vi "PC Streaming Host with slow.vi"() -> ()   [LabVIEW 2012]
uses:
  <vilib>/userdefined/High Color/nirio_resource_hc.ctl
  hv cluster control.ctl
  <vilib>/FPGAPlugInAG/PXI-7951R/niLvFpga_Open_PXI-7951R.vi
  <vilib>/rvi/interface/common/dynamic/niFpgaDynamicAddResources.vi
  <vilib>/Utility/error.llb/Error Cluster From Error Code.vi
  <vilib>/rvi/errors/niLvFpgaAdjustHostInterfaceError.vi
  <vilib>/FPGAPlugInAG/Dynamic/niLvFpga_Close_Dynamic.vi
  <vilib>/rvi/interface/nirviOpenFPGA/nirviOpenFPGA.xnode
  FPGA Bitfiles/ModuDAQ_FPGATarget_TopLevelFPGAw8LE_8T5P+CgHwo4.lvbitx
  <vilib>/rvi/interface/nirviReadWriteControl/nirviReadWriteControl.xnode
  <vilib>/rvi/interface/nirviMethod/nirviMethod.xnode
  <vilib>/rvi/interface/nirviCloseFPGA/nirviCloseFPGA.xnode
  <vilib>/ptbypt/NI_PtbyPt.lvlib
  <vilib>/rvi/interface/Simulation/niFpgaSimulationCallBeginRW.vi
  Program Files/CAEN/HV/CAENHVWrapper/labview/CAENHVWrapper/CAENHVWrapper.lvlib
  NiFpgaLv.dll
  <vilib>/FPGAPlugInAG/Dynamic/niLvFpga_ReadFifo_Dynamic.vi
  <vilib>/rvi/errors/niLvFpgaMergeErrorWithErrorCode.vi
panel:
  in  "pressed stop by user after \nfile is fully written":bool
  out "Stop after file is fully written":bool
  out "fast loop stop":bool
  in  "Channel Cluster":T1={"det_type"=["", "", "", "", "", "", "", ""], "Serial numbers"=["", "", "", "", "", "", "", ""], "Sources"=["", "", "", "", "", "", "", ""], "Trigger level"=[4000, 4000, 4000, 4000, 4000, 4000, 4000, 4000], "Data Record On/Off"=[FALSE, FALSE, FALSE, FALSE, FALSE, FALSE, FALSE, FALSE, TRUE, FALSE, FALSE, FALSE, FALSE, FALSE, FALSE, TRUE], "Number of Channels"=8}
  in  "HV Cluster":T2={"HV Power On/Off"=[TRUE, TRUE], "Set Voltage"=["0", "0", "0", "0", "0", "0", "0", "0"], "HV Tolerance (%)"=1.0}
  out "created path":path
  out "File name":string
  out "Total Data Chunks to Write":dbl
  in  "Tab Control":T3(tab)
  in  "Write mode":bool
  out "directory exists - please wait":u8(slide)
  out "directory ok":bool
  in  "Write Enable":bool
  in  "File Path":path=path "Z:/Modulation/Raw_Data/combined"
  out "File Writing Progress (%)":dbl(slide) scale=0.0..100.0
  in  "Slow Control On":bool
  in  "Fast Data On":bool
  in  "Number of Files to Write":u32=1
  in  "IP Address of NIST Time Server":string(combo)="ntp1.nikhef.nl"
  in  "VISA resource name":refnum<visa-resource-name>="COM7"
  out "HV Power On/Off":bool[](array[boolean])
  in  "HV Tolerance (%)":dbl=1.0
  out "HV(V)":sgl[](array[numeric])
  in  "IP adress HV2":string="1_0_0"
  in  "IP adress HV1":string="0_0_0"
  out "error HV":errorcluster
  out "Set Voltage":string[](array[string])=["0", "0", "0", "0", "0", "0", "0", "0"]
  out "Current(uA)":sgl[](array[numeric])
  in  "General Cluster":cluster{"Location":i16}={"Location"=1} {"Location" items=["Purdue", "NIKHEF", "Zurich", "???"]}
  in  "PXI address":T4="RIO0" caption="RIO Device"
  in  "det_type":string[](array[combo])=["NaI(Tl)", "NaI(Tl)", "NaI(Tl)", "NaI(Tl)", "NaI(Tl)", "NaI(Tl)", "NaI(Tl)", "NaI(Tl)"]
  in  "Serial numbers":string[](array[combo])=["SBJ593", "SBJ592", "SBJ590", "SBJ591", "SBJ588", "SBJ589", "SBJ586", "Other"]
  in  "Sources":string[](array[combo])=["Background", "Background", "Ti-44", "Ti-44", "Co-60", "Co-60", "Cs-137", "Cs-137"]
  in  "Trigger level":i16[](array[numeric])=[2000, 2000, 1000, 1000, 2000, 2000, 2000, 2000] caption="Trigger"
  in  "Data Record \nOn/Off":bool[](array[boolean])=[TRUE, TRUE, TRUE, TRUE, TRUE, TRUE, TRUE, TRUE]
  in  "Testpulse Cluster":T5={"Master Pulser On/Off"=FALSE, "Testpulse Turnaround Time (samples)"=14, "Pulse Separation (samples)"=0, "Pulse duration (samples)"=0}
  out "Samples per Data Chunk":u32
  in  "DAQ Info Cluster":T6={"Data Chunks per File"=1000, "Samples per Waveform"=95, "Pretrigger Samples"=15, "circular buffer length (samples)"=1000, "Waveforms per Data Chunk"=5000} {"Waveforms per Data Chunk" format="%.2p"}
  out "Average Throughput":dbl(graph)
  out "Loop Time":u32
  out "Inst. Throughput":dbl format="%#_6p"
  out "Elements in FIFO":u32(graph)
  out "FIFO Overflow":bool
  out "Current Chunk":u32
  out "Current File":i32
  out "Waveform Graph":dynamicdata(graph)
  out "Channel number displayed":i16=-1
  in  "Arduino read \nrate (Hz)":dbl=1.0
  out "Slow time":u64
  out "data":dbl[](array[numeric])
  in  "XON Character":u8=17 format="%.0x"
  in  "XOFF Character":u8=19 format="%.0x"
  out "Slow Cluster":T7
  out "read buffer":string
  out "Bad sensor?":string
  in  "Max Slow Entries per File":i32=86400
  out "Current Slow File":i32
  out "Current Slow Entry":i32
  out "Sensor out of bounds":bool
  out "Temperature":dbl(graph)
  out "Pressure":dbl(graph)
  out "magnetic field y coordinate":dbl(graph)
  out "total magnetic field":dbl(graph)
  out "magnetic field z coordinate":dbl(graph)
  out "magnetic field x coordinate":dbl(graph)
  out "humidity":dbl(graph)
  out "XML String":string
  out "Slow XML":string
  out "error out":errorcluster
  out "NIST Time":u64
  out "NIST Time Failed to Read":bool
  in  "Minutes to wait":u32=5 min=3
  out "UTC format":bool=TRUE
  out "FPGA Timestamp":u64
  out "Stopped":bool
  in  "stop":bool
  # "Channel 0"
  # "Channel 1"
  # "Channel 2"
  # "Channel 3"
  # "Channel 4"
  # "Channel 5"
  # "Channel 6"
  # "Channel 7"
  # "Write continuously"
  # "Write finite number of files"
  # "Program will stop when number of Files to Write is Complete OR if stop is pressed."
  # "These parameters are set by the set_shutdown_HV vi!"
  # "Channel 0"
  # "Channel 1"
  # "Channel 2"
  # "Channel 3"
  # "Channel 4"
  # "Channel 5"
  # "Channel 6"
  # "Channel 7"
  # "Channel 0"
  # "Channel 1"
  # "Channel 2"
  # "Channel 3"
  # "Channel 4"
  # "Channel 5"
  # "Channel 6"
  # "Channel 7"
  # "TODO: Make this look like the \"detectors\" tab"
  # "Waveform/Data Chunk information"
  # "To compare directly on a scope: Horizontal scale: 200 ns/div Vertical scale: ~100 mV/div If 15 pretriggers, delay = 700 ns"
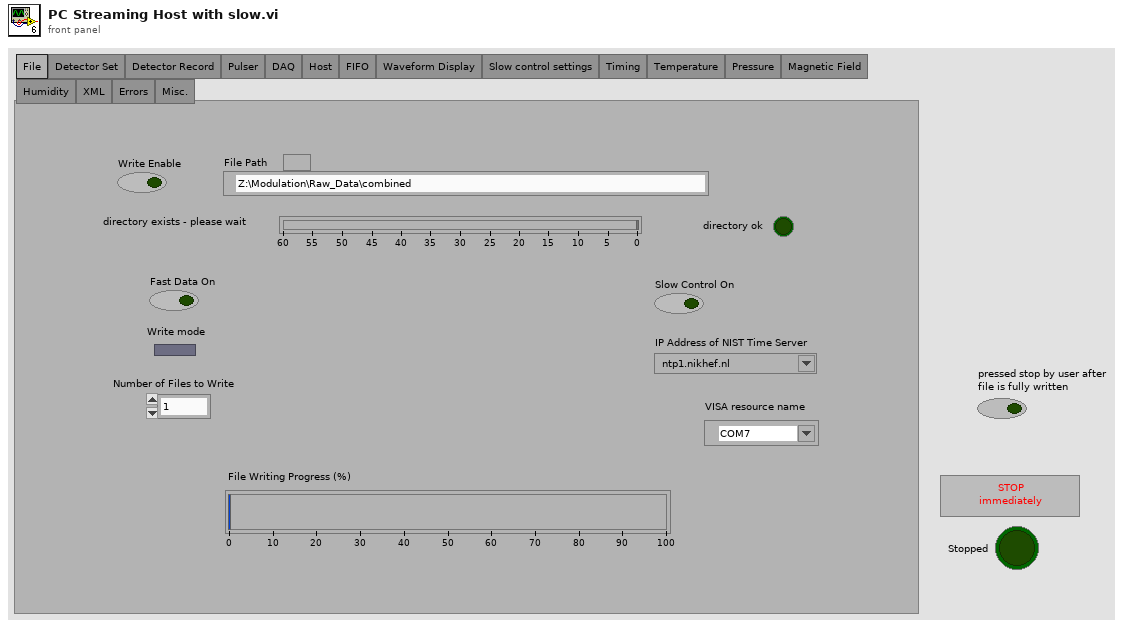
[diagram p1: front panel]
types:
  T1 = cluster{"det_type":string[], "Serial numbers":string[], "Sources":string[], "Trigger level":i16[], "Data Record On/Off":bool[], "Number of Channels":u8}
  T2 = typedef "hv cluster control.ctl" = cluster{"HV Power On/Off":bool[], "Set Voltage":string[], "HV Tolerance (%)":dbl}
  T3 = enum32{"File", "Detector Set", "Detector Record", "Pulser", "DAQ", "Host", "FIFO", "Waveform Display", "Slow control settings", "Timing", "Temperature", "Pressure", "Magnetic Field", "Humidity", "XML", "Errors", "Misc."}
  T4 = typedef "nirio_resource_hc.ctl" = tag
  T5 = cluster{"Master Pulser On/Off":bool, "Testpulse Turnaround Time (samples)":u32, "Pulse Separation (samples)":u32, "Pulse duration (samples)":u32}
  T6 = cluster{"Data Chunks per File":u32, "Samples per Waveform":u32, "Pretrigger Samples":u32, "circular buffer length (samples)":u32, "Waveforms per Data Chunk":u32}
  T7 = cluster{"Arduino \nParameters":dbl, "Total Number of \nSlow Parameters":i32, "UTC format?":bool, "Sensor Upper \nbounds":i32[], "Sensor Lower \nbounds":i32[], "Descriptions":string[], "datanames":string[]}
  T8 = cluster{"Arduino Parameters":dbl, "Total Number of Slow Parameters":i32, "UTC format?":bool, "Sensor Upper bounds":i32[], "Sensor Lower bounds":i32[], "Descriptions":string[], "datanames":string[]}
  T9 = enum16{"open", "replace", "create", "open or create", "replace or create", "replace or create with confirmation"}
  T10 = enum16{"big-endian, network order", "native, host order", "little-endian"}
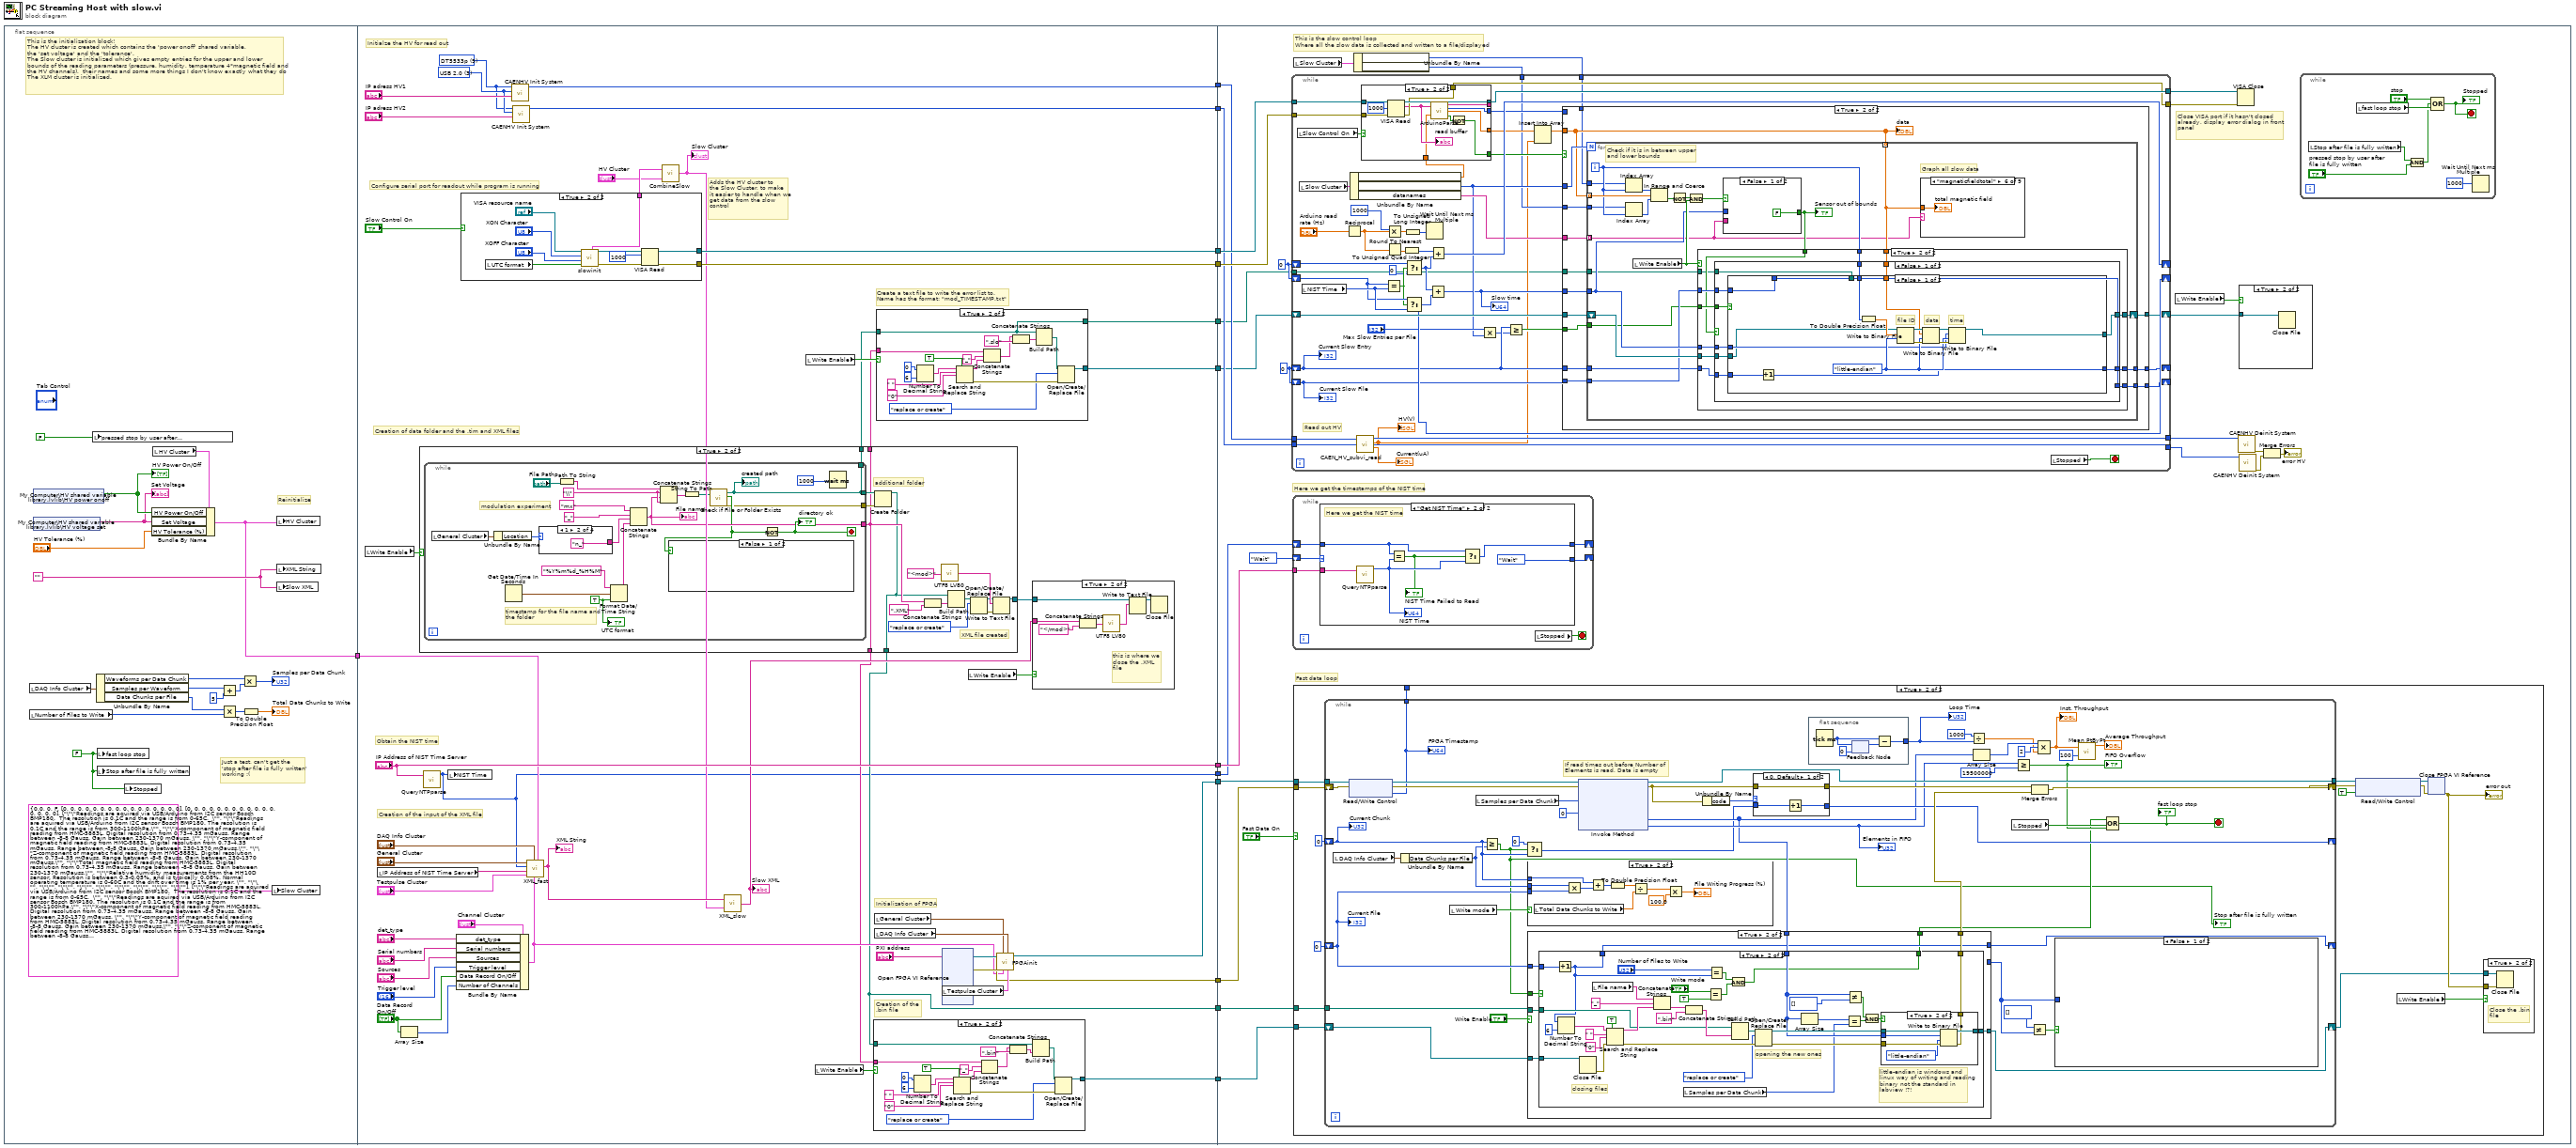
[diagram p0: block diagram]
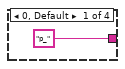
[diagram p7: hidden frame]
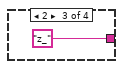
[diagram p8: hidden frame]
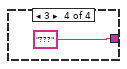
[diagram p9: hidden frame]
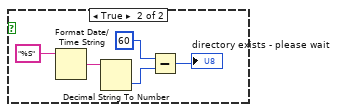
[diagram p10: hidden frame]
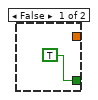
[diagram p11: hidden frame]
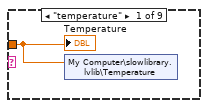
[diagram p13: hidden frame]
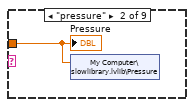
[diagram p14: hidden frame]
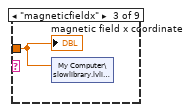
[diagram p15: hidden frame]
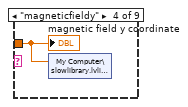
[diagram p16: hidden frame]
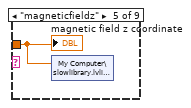
[diagram p17: hidden frame]
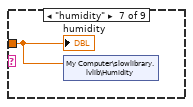
[diagram p18: hidden frame]
diagram:
  n1 = flat-sequence {
    tunnel: [w15] -> w2
    tunnel: ["IP Address of NIST Time Server"] -> w13
    tunnel: [w58] -> w12
    tunnel: [w57] -> w11
    tunnel: [w53] -> w10
    tunnel: [w52] -> w9
    tunnel: [w51] -> w8
    tunnel: [w42] -> w7
    tunnel: [w41] -> w6
    tunnel: [w40] -> w5
    tunnel: [w36] -> w4
    tunnel: [w35] -> w3
    tunnel: w2 -> [w34]
    tunnel: [w33] -> w1
    tunnel: w13 -> [w195]
    tunnel: w12 -> [w186]
    tunnel: w11 -> [w185]
    tunnel: w10 -> [w182]
    tunnel: w9 -> [w184]
    tunnel: w8 -> [w183]
    tunnel: w7 -> [w181]
    tunnel: w6 -> [w180]
    tunnel: w5 -> [w179]
    tunnel: w4 -> [w177]
    tunnel: w3 -> [w176]
    tunnel: w1 -> [w175]
    frame #0 {
      w14 = FALSE ("fast loop stop")
      w31 = ""
      # "Just a test, can't get the \n'stop after file is fully written'\nworking :("
      # "This is the initialization block!\nThe HV cluster is created which contains the 'power onoff' shared variable, \nthe 'set voltage' and the 'tolerance'.\nThe Slow cluster is initialized which gives empty entries for the upper and lower\nbounds of the reading parameters (pressure, humidity, temperature 4*magnetic field and\nthe HV channels),  their names and some more things I don't know exactly what they do\nThe XLM cluster is initialized."
      # "Reinitialize"
      n2 = local read "DAQ Info Cluster"() -> (w27:T6)
      n3 = local read "Number of Files to Write"() -> (w22:u32)
      n4 = shared-variable "My Computer\\HV shared variable library.lvlib\\HV power onoff"() -> (w17:bool[])  [unwired: 1 in, 1 out]
      "HV Power On/Off" <- w17
      n5 = shared-variable "My Computer\\HV shared variable library.lvlib\\HV voltage set"() -> (w16:string[])  [unwired: 1 in, 1 out]
      "Set Voltage" <- w16
      n6 = local write "pressed stop by user after \nfile is fully written"(FALSE ("stop 2")) -> ()
      n7 = Unbundle By Name(w27) -> ("Waveforms per Data Chunk"=w19:u32, "Samples per Waveform"=w20:u32, "Data Chunks per File"=w21:u32)
      n8 = local write "fast loop stop"(w14) -> ()
      n9 = local write "Stop after file is fully written"(w14) -> ()
      n10 = local write "Stopped"(w14) -> ()
      n11 = local read "HV Cluster"() -> (w30:T2)
      n12 = Bundle By Name(cluster=w30, "HV Power On/Off"=w17, "Set Voltage"=w16, "HV Tolerance (%)"="HV Tolerance (%)") -> (w15:T2)
      n13 = Add(x=w20, y=u32 5) -> (x+y=w24:u32)
      n14 = Multiply(x=w21, y=w22) -> (x*y=w26:u32)
      n15 = Multiply(x=w19, y=w24) -> (x*y=→"Samples per Data Chunk":u32)
      n16 = To Double Precision Float(number=w26) -> (double precision float=→"Total Data Chunks to Write":dbl)
      n17 = local write "Slow Cluster"(T8 {"Arduino Parameters"=0.0, "Total Number of Slow Parameters"=0, "UTC format?"=FALSE, "Sensor Upper bounds"=[0, 0, 0, 0, 0, 0, 0, 0, 0, 0, 0, 0, 0, 0, 0, 0], "Sensor Lower bounds"=[0, 0, 0, 0, 0, 0, 0, 0, 0, 0, 0, 0, 0, 0, 0, 0], "Descriptions"=["\"\"Readings are aquired via USB/Arduino from I2C sensor Bosch BMP180.  The resolution is 0.1C and the range is from 0-65C.  \"", "\"\"Readings are aquired via USB/Arduino from I2C sensor Bosch BMP180. The resolution is 0.1C and the range is from 300-1100hPa.\"", "\"\"X-component of magnetic field reading from HMC-5883L. Digital resolution from 0.73-4.35 mGauss. Range between -8-8 Gauss. Gain between 230-1370 mGauss. \"", "\"\"Y-component of magnetic field reading from HMC-5883L. Digital resolution from 0.73-4.35 mGauss. Range between -8-8 Gauss. Gain between 230-1370 mGauss.\"", "\"\"Z-component of magnetic field reading from HMC-5883L. Digital resolution from 0.73-4.35 mGauss. Range between -8-8 Gauss. Gain between 230-1370 mGauss.\"", "\"\"Total magnetic field reading from HMC-5883L. Digital resolution from 0.73-4.35 mGauss. Range between -8-8 Gauss. Gain between 230-1370 mGauss.\"", "\"\"Relative humidity measurements from the HH10D sensor. Resolution is between 0.3-0.05%, and is typically 0.08%. Normal operating temperature is 0-60C and the drift over time is 1% per year. \"", "\"\"", "\"\"", "\"\"", "\"\"", "\"\"", "\"\"", "\"\"", "\"\"", "\"\""], "datanames"=["\"\"Readings are aquired via USB/Arduino from I2C sensor Bosch BMP180.  The resolution is 0.1C and the range is from 0-65C.  \"", "\"\"Readings are aquired via USB/Arduino from I2C sensor Bosch BMP180. The resolution is 0.1C and the range is from 300-1100hPa.\"", "\"\"X-component of magnetic field reading from HMC-5883L. Digital resolution from 0.73-4.35 mGauss. Range between -8-8 Gauss. Gain between 230-1370 mGauss. \"", "\"\"Y-component of magnetic field reading from HMC-5883L. Digital resolution from 0.73-4.35 mGauss. Range between -8-8 Gauss. Gain between 230-1370 mGauss.\"", "\"\"Z-component of magnetic field reading from HMC-5883L. Digital resolution from 0.73-4.35 mGauss. Range between -8-8 Gauss. Gain between 230-1370 mGauss.\"", "\"\"Total magnetic field reading from HMC-5883L. Digital resolution from 0.73-4.35 mGauss. Range between -8-8 Gauss. Gain between 230-1370 mGauss.\"", "\"\"Relative humidity measurements from the HH10D sensor. Resolution is between 0.3-0.05%, and is typically 0.08%. Normal operating temperature is 0-60C and the drift over time is 1% per year. \"", "\"\"", "\"\"", "\"\"", "\"\"", "\"\"", "\"\"", "\"\"", "\"\"", "\"\""]} ("Cluster")) -> ()
      n18 = local write "HV Cluster"(w15) -> ()
      n19 = local write "XML String"(w31) -> ()
      n20 = local write "Slow XML"(w31) -> ()
    }
    frame #1 {
      w60 = 3 items=["TCP/IP"=0, "HS CAENET"=2, "USB 2.0"=3, "CONET Optical Link"=4, "USB VCP"=5] ("LinkType")
      w59 = u32 9 items=["SY1527", "SY2527", "SY4527", "SY5527", "N568", "V65XX", "N1470", "V8100", "", "DT5533p"] ("system")
      # "Creation of the \n.bin file"
      # "Obtain the NIST time"
      # "Adds the HV cluster to\nthe Slow Cluster, to make\nit easier to handle when we\nget data from the slow\ncontrol"
      # "Initialization of FPGA"
      # "Initialze the HV for read out"
      # "Create a text file to write the error list to.  \nName has the format: \"mod_TIMESTAMP.txt\""
      # "Creation of the input of the XML file"
      # "Configure serial port for readout while program is running"
      # "Creation of data folder and the .tim and XML files"
      n21 = local read "Write Enable"() -> (w81:bool)
      n22 = local read "IP Address of NIST Time Server"() -> (w72:string)
      n23 = Array Size(array="Data Record \nOn/Off") -> (size(s)=w70:i32)
      n24 = case shown="True" w81 {
        tunnel: [_ w143] -> w54
        tunnel: [_ w135] -> w56
        tunnel: [_ w133] -> w43
        tunnel: [_ w133] -> w37
        tunnel: [_ w132] -> w36
        frame False {
        }
        frame True {
          # "XML file created"
          # "additional folder"
          n25 = while {
            tunnel: [w146] -> w144
            tunnel: [w148] -> w145
            tunnel: [w148] -> w143
            tunnel: [w153] -> w133
            stop <- w158 stop-if-true
            w154 = "\\" ("string")
            w161 = TRUE ("UTC format")
            # "modulation experiment"
            # "timestamp for the file name and the folder"
            n26 = local read "General Cluster"() -> (w151:cluster{"Location":i16})
            n27 = Unbundle By Name(w151) -> ("Location"=w150:i16)
            n28 = Get Date/Time In Seconds() -> (seconds since 1Jan1904=w162:timestamp)
            n29 = case shown="1" w150 {
              tunnel: ["p_" ("string") "n_" ("string") "z_" ("string") "???"] -> w152
              frame 0, Default {
              }
              frame 1 {
              }
              frame 2 {
              }
              frame 3 {
              }
            }
            n30 = Path To String(path="File Path") -> (string=w164:string)
            n31 = Format Date/Time String(time format string (%c)="%Y%m%d_%H%M", seconds (now)=w162, UTC format=w161) -> (date/time string=w155:string)
            n32 = Concatenate Strings("mx" ("string"), "_" ("string"), w152, w155) -> (w153:string)
            "File name" <- w153
            n33 = Concatenate Strings(w164, w154, w153, w154) -> (w165:string)
            n34 = String To Path(string=w165) -> (path=w149:path)
            n35 = call <vilib>:"Check if File or Folder Exists.vi"("path"=w149) -> ("error out"=w146:errorcluster, "file or folder exists?"=w147:bool, "dup path"=w148:path)  [unwired: 8 in]
            "created path" <- w148
            n36 = case shown="False" w147 {
              frame False {
              }
              frame True {
                n37 = Format Date/Time String(time format string (%c)="%S") -> (date/time string=w173:string)  [unwired: 2 in]
                n38 = Decimal String To Number(string=w173) -> (number=w171:i32)  [unwired: 2 in, 1 out]
                n39 = Subtract(x=60, y=w171) -> (x-y=→"directory exists - please wait":i32)
              }
            }
            n40 = Not(x=w147) -> (.not. x?=w158:bool)
            "directory ok" <- w158
            n41 = Wait (ms)(milliseconds to wait=1000) -> ()  [unwired: 1 out]
            "UTC format" <- w161
          }
          n42 = Create Folder(path (use dialog)=w145, error in=w144) -> (created path=w132:path)  [unwired: 1 in, 2 out]
          n43 = Concatenate Strings(w133, ".XML" ("substring (\"\")")) -> (w139:string)
          n44 = call "UTF8 LV80.vi"("text"="<mod>") -> ("utf-8 text out"=w142:string)
          n45 = Build Path(base path=w132, name or relative path=w139) -> (appended path=w138:path)
          n46 = Open/Create/Replace File(file path (use dialog)=w138, operation (0:open)=T9."replace or create") -> (refnum out=w141:refnum<file>, error out=w140:errorcluster)  [unwired: 4 in, 1 out]
          n47 = Write to Text File(file (use dialog)=w141, text=w142, error in=w140) -> (refnum out=w135:refnum<file>)  [unwired: 1 in, 2 out]
        }
      }
      n48 = call "QueryNTPparse.vi"("IP Address of NIST Server"="IP Address of NIST Time Server") -> ("NTP Time"=w33:u64)  [unwired: 1 in, 2 out]
      n49 = local write "NIST Time"(w33) -> ()
      n50 = Bundle By Name(cluster="Channel Cluster", "det_type"="det_type", "Serial numbers"="Serial numbers", "Sources"="Sources", "Trigger level"="Trigger level", "Data Record On/Off"="Data Record \nOn/Off", "Number of Channels"=w70) -> (w39:T1)
      n51 = case shown="True" "Slow Control On" {
        tunnel: [_ w131] -> w58
        tunnel: [_ w130] -> w57
        tunnel: [_ w122] -> w80
        frame False {
        }
        frame True {
          n52 = local read "UTC format"() -> (w125:bool)
          n53 = call "slowinit.vi"("UTC format"=w125, "XOFF Character"="XOFF Character", "XON Character"="XON Character", "VISA resource name"="VISA resource name") -> ("error IO"=w123:errorcluster, "VISA resource name out"=w124:refnum<visa-resource-name>, "Slow Cluster"=w122:T8)  [unwired: 5 in]
          n54 = VISA Read(VISA resource name=w124, byte count=u32 1000, error in (no error)=w123) -> (VISA resource name out=w131:refnum<visa-resource-name>, error out=w130:errorcluster)  [unwired: 2 out]
        }
      }
      n55 = call "CAENHV Init System.vi"("Arg"="IP adress HV1", "LinkType"=w60, "system"=w59) -> ("handle"=w52:i32)  [unwired: 7 in, 1 out]
      n56 = call "CAENHV Init System.vi"("Arg"="IP adress HV2", "LinkType"=w60, "system"=w59) -> ("handle"=w51:i32)  [unwired: 7 in, 1 out]
      n57 = call "XML_fast.vi"("HV Cluster"=w34, "Channel Cluster"=w39, "DAQ Info Cluster"="DAQ Info Cluster", "Testpulse Cluster"="Testpulse Cluster", "IP Address of NIST Time Server"=w72, "NIST Time"=w33, "General Cluster"="General Cluster") -> ("XML String"=w75:string)  [unwired: 4 in]
      "XML String" <- w75
      n58 = call "CombineSlow.vi"("HV Cluster"="HV Cluster", "Slow Cluster"=w80) -> ("Slow Cluster 2"=w38:T8)
      "Slow Cluster" <- w38
      n59 = call "XML_slow.vi"("Slow Cluster"=w38, "Input String"=w75) -> ("Output String"=w76:string)
      "Slow XML" <- w76
      n60 = local read "Write Enable"() -> (w55:bool)
      n61 = local read "Write Enable"() -> (w44:bool)
      n62 = case shown="True" w44 {
        tunnel: [_ w91] -> w42
        tunnel: w37 -> [_ w83]
        tunnel: w36 -> [_ w82]
        frame False {
        }
        frame True {
          n63 = Number To Decimal String(number=0, width (-)=i16 6) -> (decimal integer string=w98:string)
          n64 = Search and Replace String(replace all?=TRUE ("replace all? (F)"), input string=w98, search string=" ", replace string="0" ("replace string (\"\")")) -> (result string=w88:string, error out=w93:errorcluster)  [unwired: 4 in, 2 out]
          n65 = Concatenate Strings(w83, "_" ("string"), w88) -> (w86:string)
          n66 = Concatenate Strings(w86, ".bin" ("substring (\"\")")) -> (w90:string)
          n67 = Build Path(base path=w82, name or relative path=w90) -> (appended path=w94:path)
          n68 = Open/Create/Replace File(file path (use dialog)=w94, error in=w93, operation (0:open)=T9."replace or create") -> (refnum out=w91:refnum<file>)  [unwired: 3 in, 2 out]
        }
      }
      n69 = local read "General Cluster"() -> (w47:cluster{"Location":i16})
      n70 = local read "DAQ Info Cluster"() -> (w48:T6)
      n71 = case shown="True" w55 {
        tunnel: [_ w108] -> w53
        tunnel: w43 -> [_ w100]
        tunnel: w54 -> [_ w99]
        tunnel: [_ w99] -> w35
        frame False {
        }
        frame True {
          n72 = Number To Decimal String(number=0, width (-)=i16 6) -> (decimal integer string=w115:string)
          n73 = Search and Replace String(replace all?=TRUE ("replace all? (F)"), input string=w115, search string=" ", replace string="0" ("replace string (\"\")")) -> (result string=w105:string, error out=w110:errorcluster)  [unwired: 4 in, 2 out]
          n74 = Concatenate Strings(w100, "_" ("string"), w105) -> (w103:string)
          n75 = Concatenate Strings(w103, ".slo" ("substring (\"\")")) -> (w107:string)
          n76 = Build Path(base path=w99, name or relative path=w107) -> (appended path=w111:path)
          n77 = Open/Create/Replace File(file path (use dialog)=w111, error in=w110, operation (0:open)=T9."replace or create") -> (refnum out=w108:refnum<file>)  [unwired: 3 in, 2 out]
        }
      }
      n78 = local read "Testpulse Cluster"() -> (w46:T5)
      n79 = xnode "Open FPGA VI Reference"("resource name"="PXI address") -> ("FPGA VI Reference Out"=w50:refnum<k20>, "error out"=w49:errorcluster)  [unwired: 1 in]
      n80 = local read "Write Enable"() -> (w63:bool)
      n81 = call "FPGAinit.vi"("Testpulse Cluster"=w46, "DAQ Info Cluster"=w48, "Channel Cluster"=w39, "General Cluster"=w47, "error in"=w49, "FPGA VI Reference In"=w50) -> ("error out"=w40:errorcluster, "FPGA VI Reference Out"=w41:refnum<k20>)  [unwired: 4 in]
      n82 = case shown="True" w63 {
        tunnel: w56 -> [_ w121]
        tunnel: w76 -> [_ w116]
        frame False {
        }
        frame True {
          # "this is where we close the .XML file"
          n83 = Concatenate Strings(w116, "</mod>" ("string")) -> (w117:string)
          n84 = call "UTF8 LV80.vi"("text"=w117) -> ("utf-8 text out"=w120:string)
          n85 = Write to Text File(file (use dialog)=w121, text=w120) -> (refnum out=w119:refnum<file>)  [unwired: 2 in, 2 out]
          n86 = Close File(refnum=w119) -> ()  [unwired: 1 in, 2 out]
        }
      }
    }
    frame #2 {
      w187 = 0
      w178 = u64 0
      # "This is the slow control loop\nWhere all the slow data is collected and written to a file/displayed"
      # "Fast data loop"
      # "Close VISA port if it hasn't closed already, display error dialog in front panel"
      # "Here we get the timestamps of the NIST time"
      n87 = while {
        shift-right: [w560] -> _
        shift-left: enum16{"Wait", "Get NIST Time", "Write"}."Wait" -> [w561]
        shift-right: [w559] -> _
        shift-left: w175 -> [w558]
        tunnel: w195 -> [w557]
        stop <- w556 stop-if-true
        n88 = case shown="\"Get NIST Time\"" w561 {
          tunnel: [w564 enum16{"Wait", "Get NIST Time", "Write"}."Wait"] -> w560
          tunnel: [w563 w579] -> w559
          tunnel: w558 -> [w563 w576]
          tunnel: w557 -> [_ w575]
          frame "Wait", Default {
            # "First we wait 'minutes to wait' and proceed with Getting the NIST time\nthis is necessary to see a  drift, if it is there, between the PFGA and NIST time"
            n89 = while {
              tunnel: [enum16{"Wait", "Get NIST Time", "Write"}."Get NIST Time"] -> w564
              tunnel: "Minutes to wait" -> [w566]
              i -> [w569]
              stop <- w570 stop-if-true
              n90 = local read "Stopped"() -> (w568:bool)
              n91 = Multiply(x=60, y=w566) -> (x*y=w565:u32)
              n92 = Wait Until Next ms Multiple(millisecond multiple=u32 1000 ("y")) -> ()  [unwired: 1 out]
              n93 = Greater Or Equal?(x=w569, y=w565) -> (x >= y?=w571:bool)
              n94 = Or(x=w571, y=w568) -> (x .or. y?=w570:bool)
            }
          }
          frame "Get NIST Time" {
            # "Here we get the NIST time"
            n95 = call "QueryNTPparse.vi"("IP Address of NIST Server"=w575) -> ("NTP Time"=w578:u64)  [unwired: 1 in, 2 out]
            "NIST Time" <- w578
            n96 = Equal?(x=w576, y=w578) -> (x = y?=w577:bool)
            "NIST Time Failed to Read" <- w577
            n97 = Select(t=w576, s=w577, f=w578) -> (s? t:f=w579:u64)
          }
        }
        n98 = local read "Stopped"() -> (w556:bool)
      }
      n99 = local read "Slow Cluster"() -> (w199:T7)
      n100 = case shown="True" "Fast Data On" {
        tunnel: [_ w402] -> _
        tunnel: w181 -> [_ w398]
        tunnel: w180 -> [_ w397]
        tunnel: w179 -> [_ w396]
        tunnel: w177 -> [_ w395]
        frame False {
        }
        frame True {
          n101 = while {
            shift-right: [w442] -> w404
            shift-left: w396 -> [w431]
            shift-right: [w438] -> _
            shift-left: u32 0 -> [w435]
            shift-right: [w423] -> _
            shift-left: 0 ("number") -> [w424]
            shift-right: [w439] -> w406
            shift-left: w398 -> [w440]
            tunnel: [w456] -> w401
            tunnel: [w428] -> w402
            tunnel: w397 -> [w417]
            tunnel: w395 -> [w415]
            stop <- w425 stop-if-true
            # "If read times out before Number of Elements is read, Data is empty"
            n102 = local read "DAQ Info Cluster"() -> (w419:T6)
            n103 = xnode "Read/Write Control"("FPGA VI Reference In"=w417, "error in"=w431) -> ("FPGA VI Reference Out"=w430:refnum<k20>, "error out"=w429:errorcluster, "Timestamp"=w428:u64)
            "FPGA Timestamp" <- w428
            n104 = Unbundle By Name(w419) -> ("Data Chunks per File"=w418:u32)
            n105 = local read "Write mode"() -> (w432:bool)
            n106 = local read "Samples per Data Chunk"() -> (w416:u32)
            n107 = Greater Or Equal?(x=w435, y=w418) -> (x >= y?=w412:bool)
            "Stop after file is fully written" <- w412
            n108 = Select(t=u32 0, s=w412, f=w435) -> (s? t:f=w414:u32)
            n109 = case shown="True" w432 {
              tunnel: w424 -> [_ w475]
              tunnel: w435 -> [_ w473]
              tunnel: w418 -> [_ w466]
              frame False {
              }
              frame True {
                n110 = local read "Total Data Chunks to Write"() -> (w470:dbl)
                n111 = Multiply(x=w466, y=w475) -> (x*y=w474:u32)
                n112 = Add(x=w473, y=w474) -> (x+y=w472:u32)
                n113 = To Double Precision Float(number=w472) -> (double precision float=w471:dbl)
                n114 = Divide(x=w471, y=w470) -> (x/y=w468:dbl)
                n115 = Multiply(x=w468, y=100.0) -> (x*y=→"File Writing Progress (%)":dbl)
              }
            }
            n116 = xnode "Invoke Method"("FPGA VI Reference In"=w430, "error in"=w429, "Number of Elements"=w416, "Timeout (ms)"=0) -> ("FPGA VI Reference Out"=w456:refnum<k20>, "error out"=w453:errorcluster, "Data"=w433:i16[], "Elements Remaining"=w434:u32)
            "Elements in FIFO" <- w434
            n117 = case shown="True" "Write Enable" {
              tunnel: w433 -> [w482 w488]
              tunnel: [w482 _] -> w422
              tunnel: w412 -> [_ w492]
              tunnel: [_ w491] -> w441
              tunnel: [w483 w490] -> w439
              tunnel: w440 -> [w483 w489]
              tunnel: w424 -> [w481 w487]
              tunnel: [w481 w486] -> w423
              tunnel: [FALSE w485] -> w413
              tunnel: w415 -> [_ w484]
              frame False {
              }
              frame True {
                n118 = case shown="True" w492 {
                  tunnel: w488 -> [w496 w521]
                  tunnel: [w495 w523] -> w491
                  tunnel: w489 -> [w500 w536]
                  tunnel: [w499 w529] -> w490
                  tunnel: w487 -> [w494 w508]
                  tunnel: [w494 w507] -> w486
                  tunnel: [FALSE w510] -> w485
                  tunnel: w484 -> [_ w509]
                  frame False {
                    # "binary writing will write 0 if there is no data"
                    n119 = Not Equal?(x=w496, y=i16[] []) -> (x != y?=w497:bool)
                    n120 = case shown="True" w497 {
                      tunnel: w500 -> [w501 w506]
                      tunnel: [w501 w505] -> w499
                      tunnel: [_ w504] -> w495
                      tunnel: w496 -> [_ w502]
                      frame False {
                      }
                      frame True {
                        n121 = Write to Binary File(file (use dialog)=w506, data=w502, 9:T10."little-endian" ("byte order (0:big-endian, network order)")) -> (refnum out=w505:refnum<file>, error out=w504:errorcluster)  [unwired: 3 in, 1 out]
                      }
                    }
                  }
                  frame True {
                    # "little-endian is windows and linux way of writing and reading binary not the standard in labview !?!"
                    # "opening the new ones"
                    # "closing files"
                    n122 = Increment(x=w508) -> (x+1=w507:i32)
                    n123 = Number To Decimal String(number=w507, width (-)=i16 6) -> (decimal integer string=w538:string)
                    n124 = Close File(refnum=w536) -> (error out=w535:errorcluster)  [unwired: 1 in, 1 out]
                    n125 = local read "File name"() -> (w517:string)
                    n126 = Search and Replace String(replace all?=TRUE ("replace all? (F)"), input string=w538, search string=" ", replace string="0" ("replace string (\"\")"), error in=w535) -> (result string=w528:string, error out=w534:errorcluster)  [unwired: 3 in, 2 out]
                    n127 = Concatenate Strings(w517, "_" ("string"), w528) -> (w524:string)
                    n128 = local read "Samples per Data Chunk"() -> (w516:u32)
                    n129 = Concatenate Strings(w524, ".bin" ("substring (\"\")")) -> (w526:string)
                    n130 = Equal?(x="Write mode", y=TRUE) -> (x = y?=w515:bool)
                    n131 = Equal?(x="Number of Files to Write", y=w507) -> (x = y?=w514:bool)
                    n132 = And(x=w514, y=w515) -> (x .and. y?=w510:bool)
                    n133 = Build Path(base path=w509, name or relative path=w526) -> (appended path=w533:path)
                    n134 = Open/Create/Replace File(file path (use dialog)=w533, error in=w534, operation (0:open)=T9."replace or create") -> (refnum out=w530:refnum<file>, error out=w531:errorcluster)  [unwired: 3 in, 1 out]
                    n135 = Array Size(array=w521) -> (size(s)=w520:i32)
                    n136 = Equal?(x=w520, y=w516) -> (x = y?=w519:bool)
                    n137 = Not Equal?(x=w521, y=i16[] []) -> (x != y?=w522:bool)
                    n138 = And(x=w522, y=w519) -> (x .and. y?=w518:bool)
                    n139 = case shown="True" w518 {
                      tunnel: w531 -> [w543 w550]
                      tunnel: w530 -> [w544 w549]
                      tunnel: [w544 w548] -> w529
                      tunnel: [w543 w547] -> w523
                      tunnel: w521 -> [_ w546]
                      frame False {
                      }
                      frame True {
                        n140 = Write to Binary File(file (use dialog)=w549, data=w546, error in=w550, 9:T10."little-endian" ("byte order (0:big-endian, network order)")) -> (refnum out=w548:refnum<file>, error out=w547:errorcluster)  [unwired: 2 in, 1 out]
                      }
                    }
                  }
                }
              }
            }
            n141 = Unbundle By Name(w453) -> ("code"=w454:i32)
            n142 = case shown="0, Default" w454 {
              tunnel: [w553 errorcluster {"status"=FALSE, "code"=0, "source"=""} ("error constant")] -> w443
              tunnel: w453 -> [w553 _]
              tunnel: w414 -> [w552 w554]
              tunnel: [w551 w554] -> w438
              frame 0, Default {
                n143 = Increment(x=w552) -> (x+1=w551:u32)
              }
              frame -50400 {
                # "Timeout"
              }
            }
            n144 = flat-sequence {
              tunnel: [w479] -> w447
              frame #0 {
                n145 = Tick Count (ms)() -> (millisecond timer value=w478:u32)
                n146 = feedback #1(u32 0 ("millisecond timer value")) -> (w477:u32)
                n147 = feedback-in #1(w478) -> ()
                n148 = Subtract(x=w478, y=w477) -> (x-y=w479:u32)
              }
            }
            n149 = Divide(x=u32 1000, y=w447) -> (x/y=w449:dbl)
            n150 = Array Size(array=w433) -> (size(s)=w452:i32)
            n151 = local read "Stopped"() -> (w427:bool)
            n152 = Greater Or Equal?(x=w434, y=u32 19500000) -> (x >= y?=w426:bool)
            "FIFO Overflow" <- w426
            n153 = Not Equal?(x=i16[] [], y=w422) -> (x != y?=w420:bool)
            n154 = Merge Errors(w443, w441) -> (w442:errorcluster)
            n155 = Compound Arithmetic op=MULTIPLY(w452, 2 ("y"), w449) -> (w446:dbl)
            "Inst. Throughput" <- w446
            n156 = case shown="False" w420 {
              tunnel: w422 -> [_ w465]
              frame False {
              }
              frame True {
                # "If Fast data isn't empty and\nno data is written to a file\nthe waveform will be plotted"
                n157 = local read "Channel Cluster"() -> (w463:T1)
                n158 = local read "General Cluster"() -> (w461:cluster{"Location":i16})
                n159 = local read "DAQ Info Cluster"() -> (w459:T6)
                n160 = Unbundle By Name(w463) -> ("Trigger level"=w462:i16[])
                n161 = Unbundle By Name(w461) -> ("Location"=w460:i16)
                n162 = Unbundle By Name(w459) -> ("Samples per Waveform"=w458:u32)
                n163 = call "displaydaqwave.vi"("Samples per Waveform"=w458, "Location"=w460, "Trigger level"=w462, "Waveform from DAQ"=w465) -> ("Waveform Graph"=→"Waveform Graph":dynamicdata, "Channel number displayed"=→"Channel number displayed":i16)  [unwired: 6 in]
              }
            }
            n164 = call <vilib>:"Mean PtByPt.vi"("x"=w446, "sample length"=100) -> ("mean"=→"Average Throughput":dbl)  [unwired: 2 in, 1 out]
            n165 = Compound Arithmetic op=OR(w413, w427, w426) -> (w425:bool)
            "fast loop stop" <- w425
            "Loop Time" <- w447
            "Current Chunk" <- w435
            "Current File" <- w424
          }
          n166 = xnode "Read/Write Control"("FPGA VI Reference In"=w401, "error in"=w404, "Stop FPGA and exit"=TRUE) -> ("FPGA VI Reference Out"=w400:refnum<k20>, "error out"=w399:errorcluster)
          n167 = local read "Write Enable"() -> (w408:bool)
          n168 = xnode "Close FPGA VI Reference"("FPGA VI Reference In"=w400, "error in"=w399) -> ("error out"=w409:errorcluster)
          "error out" <- w409
          n169 = case shown="True" w408 {
            tunnel: w409 -> [_ w410]
            tunnel: w406 -> [_ w411]
            frame False {
            }
            frame True {
              # "Close the .bin\nfile"
              n170 = Close File(refnum=w411, error in=w410) -> ()  [unwired: 2 out]
            }
          }
        }
      }
      n171 = Unbundle By Name(w199) -> ("Sensor Upper \nbounds"=w189:i32[], "Sensor Lower \nbounds"=w188:i32[])
      n172 = while {
        tunnel: [w250] -> w191
        tunnel: [w249] -> w190
        shift-right: [w242] -> _
        shift-left: w178 -> [w246]
        shift-right: [w239] -> _
        shift-left: w178 -> [w244]
        tunnel: [w208] -> w193
        tunnel: [w206] -> w192
        shift-right: [w225] -> w194
        shift-left: w182 -> [w248]
        shift-right: [w221] -> _
        shift-left: w187 -> [w222]
        shift-right: [w220] -> _
        shift-left: w187 -> [w224]
        tunnel: w189 -> [w214]
        tunnel: w188 -> [w213]
        tunnel: w186 -> [w212]
        tunnel: w185 -> [w211]
        tunnel: w184 -> [w210]
        tunnel: w183 -> [w209]
        tunnel: w176 -> [w204]
        stop <- w205 stop-if-true
        # "Read out HV"
        n173 = local read "Slow Control On"() -> (w228:bool)
        n174 = local read "Slow Cluster"() -> (w233:T7)
        n175 = local read "NIST Time"() -> (w247:u64)
        n176 = Reciprocal(x="Arduino read \nrate (Hz)") -> (1/x=w236:dbl)
        n177 = Unbundle By Name(w233) -> ("Arduino \nParameters"=w229:dbl, "Total Number of \nSlow Parameters"=w218:i32, "datanames"=w226:string[])
        n178 = call "CAEN_HV_subvi_read.vi"("handle HV1"=w210, "handle HV2"=w209) -> ("handle HV1 out"=w208:i32, "HV"=w207:sgl[], "Current"=→"Current(uA)":sgl[], "handle HV2 out"=w206:i32)  [unwired: 1 in, 1 out]
        "HV(V)" <- w207
        n179 = case shown="True" w228 {
          tunnel: [_ w262] -> w250
          tunnel: [_ w261] -> w249
          tunnel: [_ w259] -> w232
          tunnel: [_ w258] -> _
          tunnel: [TRUE w254] -> w227
          tunnel: [_ w256] -> w231
          tunnel: w229 -> [_ w255]
          tunnel: w212 -> [_ w253]
          tunnel: w211 -> [_ w252]
          frame False {
          }
          frame True {
            n180 = VISA Read(VISA resource name=w253, byte count=u32 1000, error in (no error)=w252) -> (VISA resource name out=w262:refnum<visa-resource-name>, read buffer=w260:string, error out=w261:errorcluster)  [unwired: 1 out]
            "read buffer" <- w260
            n181 = call "ArduinoParse.vi"("read buffer"=w260, "Expected Arduino Parameters"=w255) -> ("Number Arduino Parameters"=w259:i32, "Arduino Data Names"=w258:string[], "Arduino Data"=w256:dbl[], "Arduino Read Failed?"=w257:bool)
            n182 = Not(x=w257) -> (.not. x?=w254:bool)
          }
        }
        n183 = Equal?(x=w246, y=w247) -> (x = y?=w245:bool)
        n184 = Multiply(x=u32 1000 ("millisecond multiple"), y=w236) -> (x*y=w238:dbl)
        n185 = Round To Nearest(number=w236) -> (nearest integer value=w235:dbl)
        n186 = To Unsigned Quad Integer(1:w235) -> (0:w234:u64)
        n187 = To Unsigned Long Integer(number=w238) -> (unsigned 32bit integer=w237:u32)
        n188 = Select(t=w244, s=w245, f=0) -> (s? t:f=w240:u64)
        n189 = Select(t=w246, s=w245, f=w247) -> (s? t:f=w242:u64)
        n190 = Wait Until Next ms Multiple(millisecond multiple=w237) -> ()  [unwired: 1 out]
        n191 = Add(x=w240, y=w242) -> (x+y=w215:u64)
        "Slow time" <- w215
        n192 = Add(x=w234, y=w240) -> (x+y=w239:u64)
        n193 = Multiply(x="Max Slow Entries per File", y=w218) -> (x*y=w217:i32)
        n194 = Greater Or Equal?(x=w222, y=w217) -> (x >= y?=w223:bool)
        n195 = Insert Into Array(array=w231, new element=w207) -> (w230:dbl[])  [unwired: 1 in]
        n196 = case shown="True" w227 {
          tunnel: w248 -> [w266 w280]
          tunnel: w215 -> [_ w279]
          tunnel: [w266 w276] -> w225
          tunnel: w232 -> [_ _]
          tunnel: w230 -> [_ w270]
          tunnel: w226 -> [_ w278]
          tunnel: w218 -> [_ w277]
          tunnel: w224 -> [w264 w275]
          tunnel: w223 -> [_ w274]
          tunnel: w222 -> [w265 w273]
          tunnel: [w265 w272] -> w221
          tunnel: [w264 w271] -> w220
          tunnel: w214 -> [_ w269]
          tunnel: w213 -> [_ w268]
          tunnel: w204 -> [_ w267]
          frame False {
          }
          frame True {
            n197 = for {
              N: w277 -> [_]
              tunnel: w279 -> [w298]
              tunnel: w270 -> [w301] mode=indexing
              tunnel: w278 -> [w286] mode=indexing
              tunnel: w270 -> [w287] mode=indexing
              tunnel: w275 -> [w295]
              tunnel: w274 -> [w293]
              tunnel: w273 -> [w292]
              tunnel: [w291] -> w272
              tunnel: [w290] -> w271
              shift-right: [w296] -> w276
              shift-left: w280 -> [w297]
              tunnel: w269 -> [w285]
              tunnel: w268 -> [w284]
              tunnel: w267 -> [w281]
              i -> [w294]
              # "Check if it is in between upper \nand lower bounds"
              # "Graph all slow data"
              n198 = Index Array(array=w285, index=w294) -> (element=w282:i32)
              n199 = Index Array(array=w284, index=w294) -> (element=w283:i32)
              n200 = local read "Write Enable"() -> (w299:bool)
              n201 = In Range and Coerce(upper limit=w282, x=w301, lower limit=w283) -> (In Range?=w289:bool)  [unwired: 1 out]
              n202 = Not(x=w289) -> (.not. x?=w302:bool)
              n203 = And(x=w302, y=w299) -> (x .and. y?=w300:bool)
              n204 = case shown="False" w300 {
                tunnel: w286 -> [_ w385]
                tunnel: w298 -> [_ _]
                tunnel: [FALSE ("Sensor out of bounds") TRUE ("Sensor out of bounds")] -> w288
                frame False {
                }
                frame True {
                  "Bad sensor?" <- w385
                }
              }
              "Sensor out of bounds" <- w288
              n205 = case shown="True" w299 {
                tunnel: [w310 w324] -> w290
                tunnel: w287 -> [_ w323]
                tunnel: w298 -> [_ w322]
                tunnel: w297 -> [w312 w321]
                tunnel: [w312 w320] -> w296
                tunnel: w295 -> [w310 w319]
                tunnel: w294 -> [_ w318]
                tunnel: w293 -> [_ w317]
                tunnel: w292 -> [w311 w316]
                tunnel: [w311 w315] -> w291
                tunnel: w288 -> [_ w314]
                tunnel: w281 -> [_ w313]
                frame False {
                }
                frame True {
                  n206 = case shown="False" w314 {
                    tunnel: [w335 w382] -> w324
                    tunnel: w323 -> [w334 _]
                    tunnel: w322 -> [w333 _]
                    tunnel: w321 -> [w332 w381]
                    tunnel: [w331 w381] -> w320
                    tunnel: w319 -> [w330 w382]
                    tunnel: w318 -> [w329 _]
                    tunnel: w317 -> [w328 _]
                    tunnel: w316 -> [w327 w383]
                    tunnel: [w326 w383] -> w315
                    tunnel: w313 -> [w325 _]
                    frame False {
                      n207 = case shown="False" w328 {
                        tunnel: [w339 w352] -> w335
                        tunnel: w334 -> [w343 w360]
                        tunnel: w333 -> [w342 w359]
                        tunnel: w332 -> [w340 w358]
                        tunnel: [w341 w356] -> w331
                        tunnel: w330 -> [w339 w355]
                        tunnel: w329 -> [w338 w354]
                        tunnel: w327 -> [w337 _]
                        tunnel: [w336 0] -> w326
                        tunnel: w325 -> [_ w350]
                        frame False {
                          w344 = T10."little-endian" ("byte order (0:big-endian, network order)")
                          # "time"
                          # "data"
                          # "file ID"
                          n208 = Increment(x=w337) -> (x+1=w336:i32)
                          n209 = To Double Precision Float(number=w338) -> (double precision float=w345:dbl)
                          n210 = Write to Binary File(file (use dialog)=w340, data=w345, 9:w344) -> (refnum out=w348:refnum<file>, error out=w349:errorcluster)  [unwired: 3 in, 1 out]
                          n211 = Write to Binary File(file (use dialog)=w348, data=w343, error in=w349, 9:w344) -> (refnum out=w347:refnum<file>, error out=w346:errorcluster)  [unwired: 2 in, 1 out]
                          n212 = Write to Binary File(file (use dialog)=w347, data=w342, error in=w346, 9:w344) -> (refnum out=w341:refnum<file>)  [unwired: 2 in, 2 out]
                        }
                        frame True {
                          w361 = T10."little-endian" ("byte order (0:big-endian, network order)")
                          w351 = TRUE ("replace all? (F)")
                          # "time"
                          # "data"
                          # "file ID"
                          # "opening the new ones"
                          # "closing files"
                          n213 = Increment(x=w355) -> (x+1=w352:i32)
                          n214 = Number To Decimal String(number=w352, width (-)=i16 6) -> (decimal integer string=w377:string)
                          n215 = Close File(refnum=w358) -> (error out=w375:errorcluster)  [unwired: 1 in, 1 out]
                          n216 = local read "File name"() -> (w367:string)
                          n217 = Search and Replace String(replace all?=w351, case sensitive?=w351, input string=w377, search string=" ", replace string="0" ("replace string (\"\")"), error in=w375) -> (result string=w371:string, error out=w374:errorcluster)  [unwired: 2 in, 2 out]
                          n218 = Concatenate Strings(w367, "_" ("string"), w371) -> (w368:string)
                          n219 = Concatenate Strings(w368, ".slo" ("substring (\"\")")) -> (w369:string)
                          n220 = Build Path(base path=w350, name or relative path=w369) -> (appended path=w373:path)
                          n221 = Open/Create/Replace File(file path (use dialog)=w373, error in=w374, operation (0:open)=T9."replace or create") -> (refnum out=w357:refnum<file>)  [unwired: 3 in, 2 out]
                          n222 = To Double Precision Float(number=w354) -> (double precision float=w362:dbl)
                          n223 = Write to Binary File(file (use dialog)=w357, data=w362, 9:w361) -> (refnum out=w365:refnum<file>, error out=w366:errorcluster)  [unwired: 3 in, 1 out]
                          n224 = Write to Binary File(file (use dialog)=w365, data=w360, error in=w366, 9:w361) -> (refnum out=w364:refnum<file>, error out=w363:errorcluster)  [unwired: 2 in, 1 out]
                          n225 = Write to Binary File(file (use dialog)=w364, data=w359, error in=w363, 9:w361) -> (refnum out=w356:refnum<file>)  [unwired: 2 in, 2 out]
                        }
                      }
                    }
                    frame True {
                    }
                  }
                }
              }
              n226 = case shown="\"magneticfieldtotal\"" w286 {
                tunnel: w287 -> [w303 w304 w305 w306 w307 w308 w309 _ _]
                frame "temperature" {
                  n227 = shared-variable "My Computer\\slowlibrary.lvlib\\Temperature"(w303) -> ()  [unwired: 1 in, 1 out]
                  "Temperature" <- w303
                }
                frame "pressure" {
                  n228 = shared-variable "My Computer\\slowlibrary.lvlib\\Pressure"(w304) -> ()  [unwired: 1 in, 1 out]
                  "Pressure" <- w304
                }
                frame "magneticfieldx" {
                  n229 = shared-variable "My Computer\\slowlibrary.lvlib\\B_x"(w305) -> ()  [unwired: 1 in, 1 out]
                  "magnetic field x coordinate" <- w305
                }
                frame "magneticfieldy" {
                  n230 = shared-variable "My Computer\\slowlibrary.lvlib\\B_y"(w306) -> ()  [unwired: 1 in, 1 out]
                  "magnetic field y coordinate" <- w306
                }
                frame "magneticfieldz" {
                  n231 = shared-variable "My Computer\\slowlibrary.lvlib\\B_z"(w307) -> ()  [unwired: 1 in, 1 out]
                  "magnetic field z coordinate" <- w307
                }
                frame "magneticfieldtotal" {
                  "total magnetic field" <- w308
                }
                frame "humidity" {
                  n232 = shared-variable "My Computer\\slowlibrary.lvlib\\Humidity"(w309) -> ()  [unwired: 1 in, 1 out]
                  "humidity" <- w309
                }
                frame "seconds" {
                }
                frame "", Default {
                }
              }
            }
            "data" <- w270
          }
        }
        n233 = local read "Stopped"() -> (w205:bool)
        "Current Slow Entry" <- w222
        "Current Slow File" <- w224
      }
      n234 = local read "Write Enable"() -> (w200:bool)
      n235 = VISA Close(VISA resource name=w191, error in (no error)=w190) -> ()  [unwired: 1 out]
      n236 = call "CAENHV Deinit System.vi"("handle"=w193) -> ("error out"=w198:errorcluster)  [unwired: 10 in]
      n237 = case shown="True" w200 {
        tunnel: w194 -> [_ w387]
        frame False {
        }
        frame True {
          n238 = Close File(refnum=w387) -> ()  [unwired: 1 in, 2 out]
        }
      }
      n239 = call "CAENHV Deinit System.vi"("handle"=w192) -> ("error out"=w197:errorcluster)  [unwired: 10 in]
      n240 = Merge Errors(w198, w197) -> (→"error HV":errorcluster)
      n241 = while {
        stop <- w392 stop-if-true
        n242 = local read "Stop after file is fully written"() -> (w390:bool)
        n243 = local read "fast loop stop"() -> (w391:bool)
        n244 = Compound Arithmetic op=AND(w390, "pressed stop by user after \nfile is fully written") -> (w389:bool)
        n245 = Compound Arithmetic op=OR("stop", w389, w391) -> (w392:bool)
        "Stopped" <- w392
        n246 = Wait Until Next ms Multiple(millisecond multiple=u32 1000 ("y")) -> ()  [unwired: 1 out]
      }
    }
  }
